vi "MoveRotationMount Template.vi"(6 "HWSerialNum":i32, 7 "error in (no error)":errorcluster, 9 "DesiredAngle":sgl=320.0, 10 "Mode":T1(ring)) -> (0 "final error out":errorcluster, 1 "FinalAngle":sgl, 3 "Elapsed Time (s)":dbl)   [LabVIEW 2013]
panel:
  in  "tolerance":sgl=0.01
  out "GetStatusBits_Bits at start":i32 format="%b"
  out "GetStatusBits_Bits continual":i32 format="%b"
  out "CurrentAngle":sgl
  in  "PumpHWP":refnum<k7>(container)
  # "To see whether or not device is moving, look at the last 8 bits of the output from the method\n'GetStatusBits_Bits'\n\nIf the last 8 bits is = 0, then it's no longer moving! (that's when you stop!)"
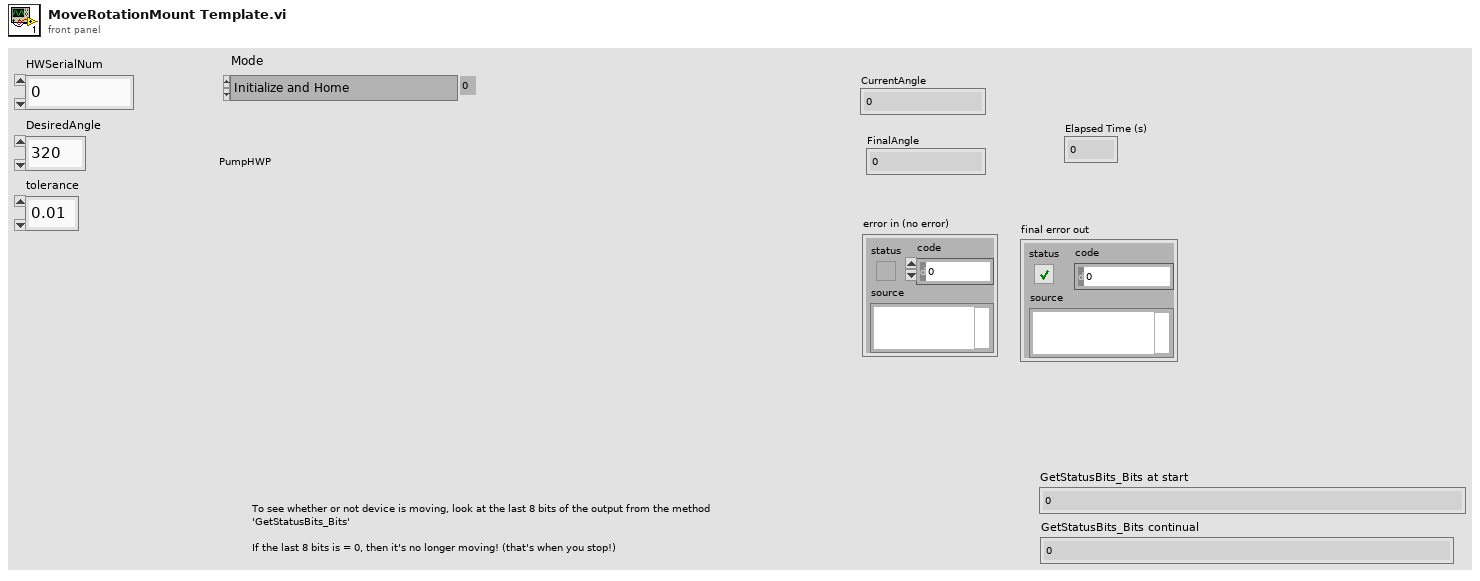
[diagram p1: front panel]
types:
  T1 = enum16{"Initialize and Home", "Move to an Angle", "Read Current Angle only", "StopCtrl"}
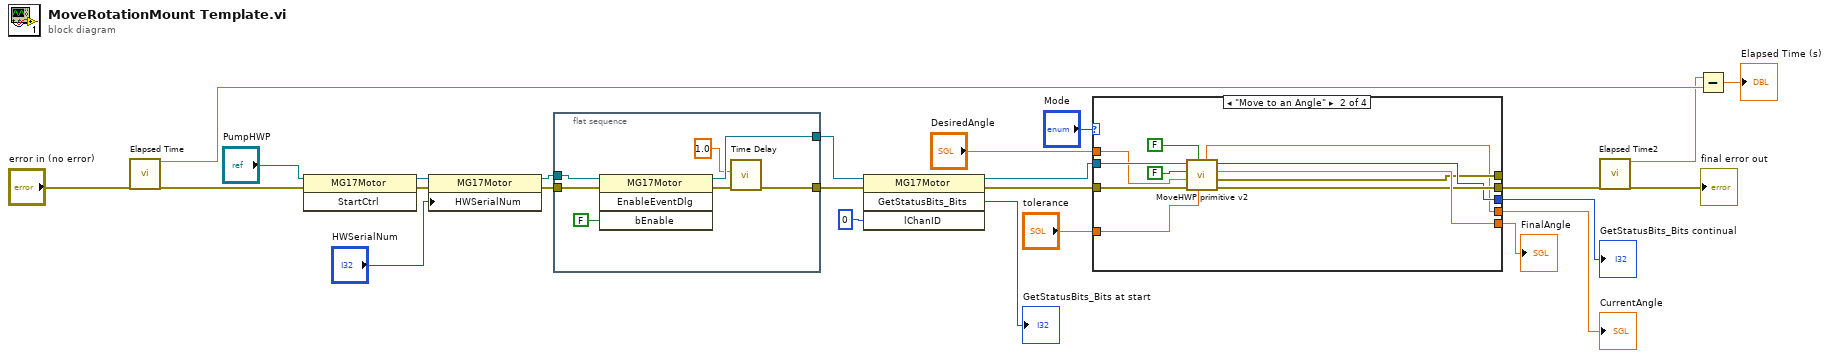
[diagram p0: block diagram]
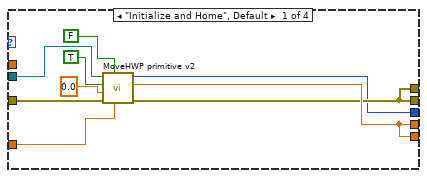
[diagram p2: hidden frame]
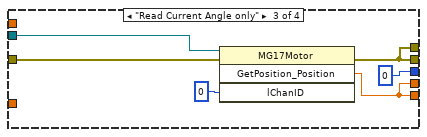
[diagram p3: hidden frame]
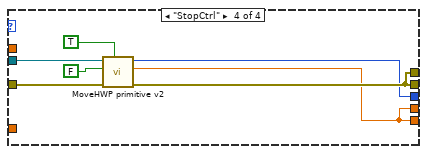
[diagram p4: hidden frame]
diagram:
  n1 = call "Elapsed Time"("error in (no error)"="error in (no error)") -> ("Present (s)"=w21:dbl, "error out"=w22:errorcluster)  [unwired: 11 in, 6 out]
  n2 = invoke class="MG17Motor" method="StartCtrl"(reference="PumpHWP", error in=w22) -> (reference out=w24:refnum<k7>, error out=w25:errorcluster)  [unwired: 1 in, 1 out]
  n3 = property class="MG17Motor"(reference=w24, error in=w25, "HWSerialNum"="HWSerialNum") -> (reference out=w7:refnum<k7>, error out=w6:errorcluster)
  n4 = flat-sequence {
    tunnel: w7 -> [w31]
    tunnel: w6 -> [w30]
    tunnel: [w27] -> w5
    tunnel: [w29] -> w4
    frame #0 {
      n5 = invoke class="MG17Motor" method="EnableEventDlg"(reference=w31, error in=w30, "bEnable"=FALSE) -> (reference out=w29:refnum<k7>, error out=w28:errorcluster)  [unwired: 1 in, 2 out]
      n6 = call "Time Delay"("error in (no error)"=w28, "Delay Time (s)"=1.0) -> ("error out"=w27:errorcluster)  [unwired: 9 in]
    }
  }
  n7 = invoke class="MG17Motor" method="GetStatusBits_Bits"(reference=w4, error in=w5, "lChanID"=0) -> (reference out=w13:refnum<k7>, error out=w12:errorcluster, "GetStatusBits_Bits"=→"GetStatusBits_Bits at start":i32)  [unwired: 1 in, 1 out]
  n8 = case shown="\"Move to an Angle\"" "Mode" {
    tunnel: [w37 w52 w55 w60] -> w19
    tunnel: [w36 w51 w54 w65] -> w18
    tunnel: w13 -> [w41 w50 w57 w64]
    tunnel: w12 -> [w39 w49 w58 w63]
    tunnel: "tolerance" -> [w33 w48 _ _]
    tunnel: [w35 w47 0 ("GetStatusBits_Bits continual") w59] -> w9
    tunnel: [w36 w46 w54 w65] -> _
    tunnel: [w37 w45 w55 w60] -> w8
    tunnel: "DesiredAngle" -> [_ w43 _ _]
    frame "Initialize and Home", Default {
      n9 = call "MoveHWP primitive v2.vi"("tolerance"=w33, "StopCtrl"=FALSE, "error in (no error)"=w39, "DesiredAngle"=sgl 0.0, "HomeTheStage"=TRUE, "Automation Refnum in"=w41) -> ("error out"=w36:errorcluster, "GetPosition_Position"=w37:sgl, "GetStatusBits_Bits continual"=w35:i32)  [unwired: 1 in, 2 out]
    }
    frame "Move to an Angle" {
      n10 = call "MoveHWP primitive v2.vi"("tolerance"=w48, "StopCtrl"=FALSE, "error in (no error)"=w49, "DesiredAngle"=w43, "HomeTheStage"=FALSE, "Automation Refnum in"=w50) -> ("error out"=w51:errorcluster, "running error out"=w46:errorcluster, "GetPosition_Position"=w52:sgl, "GetStatusBits_Bits continual"=w47:i32, "CurrentAngle"=w45:sgl)  [unwired: 1 in]
    }
    frame "Read Current Angle only" {
      n11 = invoke class="MG17Motor" method="GetPosition_Position"(reference=w57, error in=w58, "lChanID"=0) -> (error out=w54:errorcluster, "GetPosition_Position"=w55:sgl)  [unwired: 1 in, 2 out]
    }
    frame "StopCtrl" {
      n12 = call "MoveHWP primitive v2.vi"("StopCtrl"=TRUE, "error in (no error)"=w63, "HomeTheStage"=FALSE, "Automation Refnum in"=w64) -> ("error out"=w65:errorcluster, "GetPosition_Position"=w60:sgl, "GetStatusBits_Bits continual"=w59:i32)  [unwired: 3 in, 2 out]
    }
  }
  "FinalAngle" <- w19
  "GetStatusBits_Bits continual" <- w9
  "CurrentAngle" <- w8
  n13 = call "Elapsed Time2"("error in (no error)"=w18) -> ("Present (s)"=w16:dbl, "error out"=→"final error out":errorcluster)  [unwired: 11 in, 6 out]
  n14 = Subtract(x=w16, y=w21) -> (x-y=→"Elapsed Time (s)":dbl)
